vi "motor_all_shut_down.vi"(8 "error in":errorcluster, 11 "Modbus master in":refnum<class "Modbus Master.lvclass">) -> (0 "error out":errorcluster, 3 "Modbus master out":refnum<class "Modbus Master.lvclass">)   [LabVIEW 2020]
uses:
  <vilib>/NI/Modbus Library/API/Master/Modbus Master.lvclass
  C:/Program Files/National Instruments/LabVIEW 2020/vi.lib/NI/Modbus Library/API/Modbus API.lvclass
  <vilib>/NI/Modbus Library/API/Modbus API.lvclass/Modbus API.ctl
  <vilib>/NI/Modbus Library/Transmission Data Unit/Transmission Data Unit.lvclass/Transmission Data Unit.ctl
  <vilib>/NI/Modbus Library/Transmission Data Unit/Write Unit ID.vi
  <vilib>/NI/Modbus Library/API/Read Transmission Data Unit.vi
  <vilib>/NI/Modbus Library/API/Write Transmission Data Unit.vi
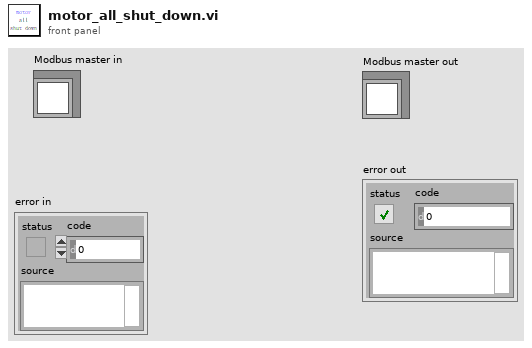
[diagram p1: front panel]
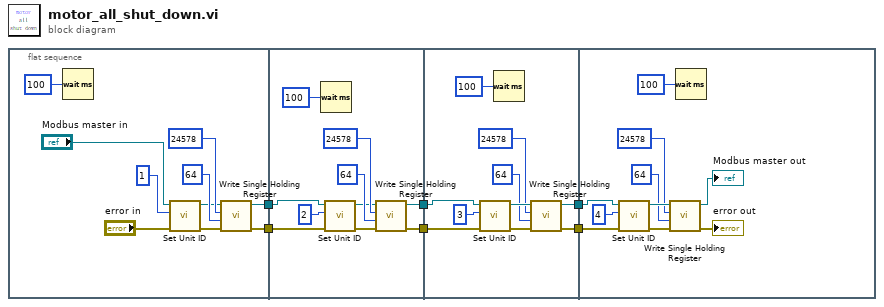
[diagram p0: block diagram]
diagram:
  n1 = flat-sequence {
    tunnel: [w9] -> w6
    tunnel: [w8] -> w5
    tunnel: w6 -> [w20]
    tunnel: w5 -> [w21]
    tunnel: [w19] -> w2
    tunnel: [w18] -> w1
    tunnel: [w31] -> w4
    tunnel: [w30] -> w3
    tunnel: w2 -> [w29]
    tunnel: w1 -> [w28]
    tunnel: w4 -> [w39]
    tunnel: w3 -> [w38]
    frame #0 {
      n2 = Wait (ms)(milliseconds to wait=u32 100) -> ()  [unwired: 1 out]
      n3 = call <vilib>:"Set Unit ID.vi"("error in"="error in", "unit ID"=u8 1, "Modbus master in"="Modbus master in") -> ("error out"=w11:errorcluster, "Modbus master out"=w12:refnum<class "Modbus Master.lvclass">)  [unwired: 7 in]
      n4 = call-dynamic "Write Single Holding Register.vi"("error in"=w11, "register to write"=u16 64 ("address"), "address"=u16 24578, "Modbus master in"=w12) -> ("error out"=w9:errorcluster, "Modbus master out"=w8:refnum<class "Modbus Master.lvclass">)  [unwired: 6 in]
    }
    frame #1 {
      n5 = Wait (ms)(milliseconds to wait=u32 100) -> ()  [unwired: 1 out]
      n6 = call <vilib>:"Set Unit ID.vi"("error in"=w20, "unit ID"=u8 2, "Modbus master in"=w21) -> ("error out"=w23:errorcluster, "Modbus master out"=w24:refnum<class "Modbus Master.lvclass">)  [unwired: 7 in]
      n7 = call-dynamic "Write Single Holding Register.vi"("error in"=w23, "register to write"=u16 64 ("address"), "address"=u16 24578, "Modbus master in"=w24) -> ("error out"=w18:errorcluster, "Modbus master out"=w19:refnum<class "Modbus Master.lvclass">)  [unwired: 6 in]
    }
    frame #2 {
      n8 = call <vilib>:"Set Unit ID.vi"("error in"=w28, "unit ID"=u8 3, "Modbus master in"=w29) -> ("error out"=w35:errorcluster, "Modbus master out"=w36:refnum<class "Modbus Master.lvclass">)  [unwired: 7 in]
      n9 = Wait (ms)(milliseconds to wait=u32 100) -> ()  [unwired: 1 out]
      n10 = call-dynamic "Write Single Holding Register.vi"("error in"=w35, "register to write"=u16 64 ("address"), "address"=u16 24578, "Modbus master in"=w36) -> ("error out"=w30:errorcluster, "Modbus master out"=w31:refnum<class "Modbus Master.lvclass">)  [unwired: 6 in]
    }
    frame #3 {
      n11 = call <vilib>:"Set Unit ID.vi"("error in"=w38, "unit ID"=u8 4, "Modbus master in"=w39) -> ("error out"=w45:errorcluster, "Modbus master out"=w46:refnum<class "Modbus Master.lvclass">)  [unwired: 7 in]
      n12 = call-dynamic "Write Single Holding Register.vi"("error in"=w45, "register to write"=u16 64 ("address"), "address"=u16 24578, "Modbus master in"=w46) -> ("error out"=→"error out":errorcluster, "Modbus master out"=→"Modbus master out":refnum<class "Modbus Master.lvclass">)  [unwired: 6 in]
      n13 = Wait (ms)(milliseconds to wait=u32 100) -> ()  [unwired: 1 out]
    }
  }
